vi "AutoRotate.vi"(9 "AccelRate":dbl, 10 "Actual":dbl, 11 "Desired":dbl) -> (3 "Right":dbl)   [LabVIEW 2013]
doc: "The quickest and most efficient algorithm for automatically rotating the robot to a given orientation. Remember, winners us this VI."
panel:
  out "Left":dbl
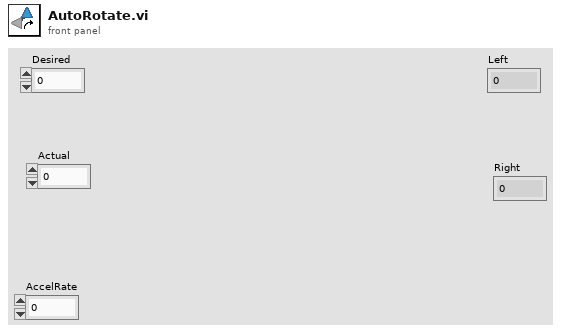
[diagram p1: front panel]
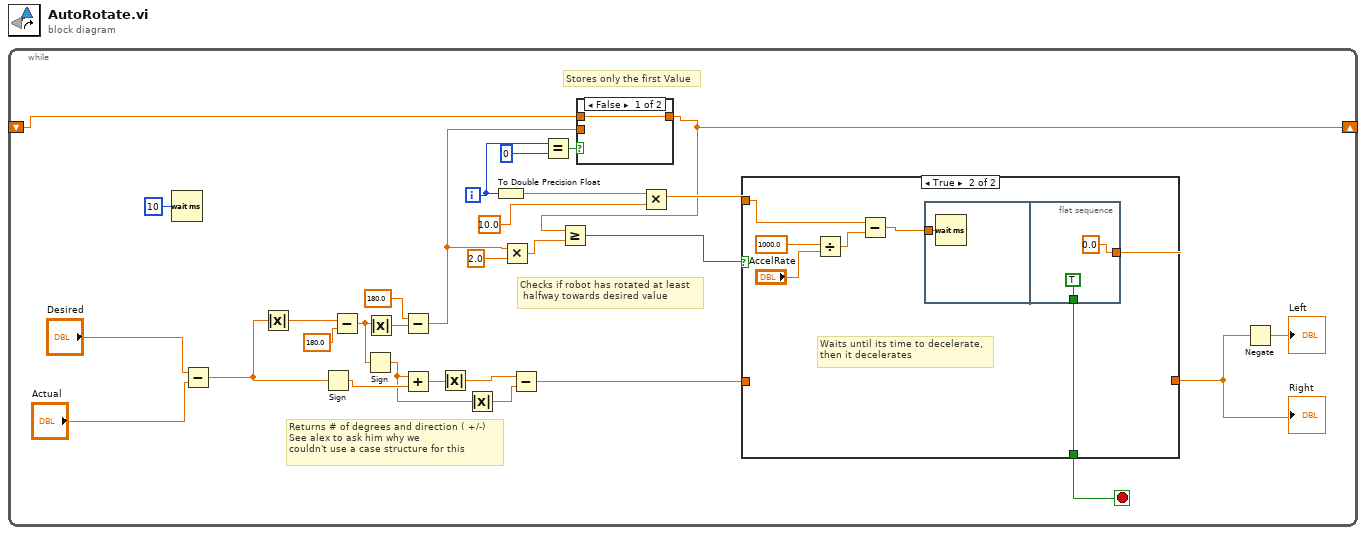
[diagram p0: block diagram]
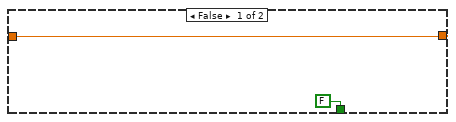
[diagram p3: hidden frame]
diagram:
  n1 = while {
    shift-right: [w10] -> _
    shift-left: _ -> [w11]
    i -> [w14]
    stop <- w16 stop-if-true
    # "Stores only the first Value"
    # "Checks if robot has rotated at least\n halfway towards desired value"
    # "Returns # of degrees and direction ( +/-)\nSee alex to ask him why we \ncouldn't use a case structure for this"
    n2 = Wait (ms)(milliseconds to wait=u32 10) -> ()  [unwired: 1 out]
    n3 = Subtract(x="Desired", y="Actual") -> (x-y=w29:dbl)
    n4 = Absolute Value(x=w29) -> (abs(x)=w28:dbl)
    n5 = Sign(1:w29) -> (0:w6:dbl)
    n6 = Subtract(x=w28, y=180.0) -> (x-y=w23:dbl)
    n7 = Sign(1:w23) -> (0:w2:dbl)
    n8 = Absolute Value(x=w23) -> (abs(x)=w26:dbl)
    n9 = Subtract(x=180.0, y=w26) -> (x-y=w8:dbl)
    n10 = Add(x=w2, y=w6) -> (x+y=w5:dbl)
    n11 = Absolute Value(x=w5) -> (abs(x)=w4:dbl)
    n12 = Absolute Value(x=w2) -> (abs(x)=w3:dbl)
    n13 = To Double Precision Float(number=w14) -> (double precision float=w19:dbl)
    n14 = Multiply(x=w8, y=2.0) -> (x*y=w9:dbl)
    n15 = Subtract(x=w4, y=w3) -> (x-y=w1:dbl)
    n16 = Equal?(x=w14, y=0) -> (x = y?=w13:bool)
    n17 = case shown="False" w13 {
      tunnel: w8 -> [_ w32]
      tunnel: w11 -> [w31 _]
      tunnel: [w31 w32] -> w10
      frame False {
      }
      frame True {
      }
    }
    n18 = Greater Or Equal?(x=w10, y=w9) -> (x >= y?=w12:bool)
    n19 = Multiply(x=w19, y=10.0) -> (x*y=w17:dbl)
    n20 = case shown="True" w12 {
      tunnel: [w33 w36] -> w20
      tunnel: w17 -> [_ w38]
      tunnel: [FALSE w35] -> w16
      tunnel: w1 -> [w33 _]
      frame False {
      }
      frame True {
        # "Waits until its time to decelerate,\nthen it decelerates"
        n21 = Divide(x=1000.0, y="AccelRate") -> (x/y=w39:dbl)
        n22 = Subtract(x=w38, y=w39) -> (x-y=w37:dbl)
        n23 = flat-sequence {
          tunnel: w37 -> [w42]
          tunnel: [0.0] -> w36
          tunnel: [TRUE] -> w35
          frame #0 {
            n24 = Wait (ms)(milliseconds to wait=w42) -> ()  [unwired: 1 out]
          }
          frame #1 {
          }
        }
      }
    }
    "Right" <- w20
    n25 = Negate(x=w20) -> (-x=→"Left":dbl)
  }
